vi "ConfigFlattenProgramToXML.vi"(8 "error in (no error)":errorcluster, 11 "ProgramArray":string[][](array[string])) -> (0 "error out":errorcluster, 3 "ProgramXML":string)   [LabVIEW 2018, in "Config.lvlib"]
uses:
  Config.lvlib
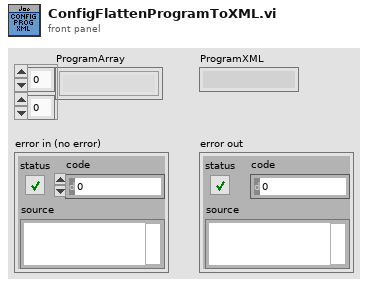
[diagram p1: front panel]
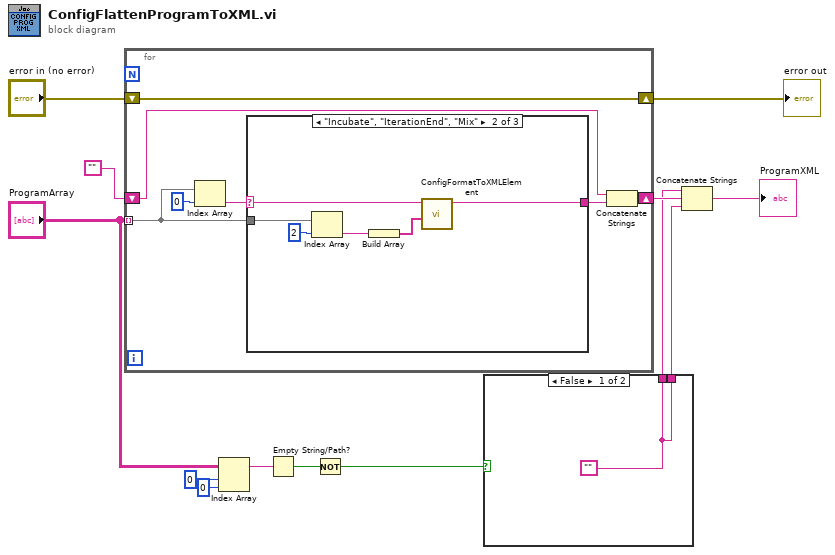
[diagram p0: block diagram]
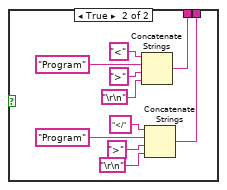
[diagram p2: hidden frame]
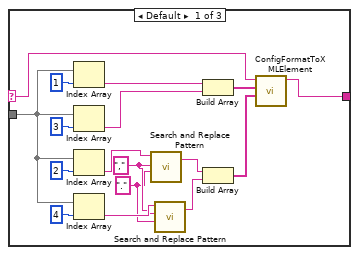
[diagram p3: hidden frame]
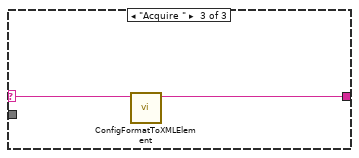
[diagram p4: hidden frame]
diagram:
  n1 = for {
    tunnel: "ProgramArray" -> [w18] mode=indexing
    shift-right: [w16] -> w10
    shift-left: "" -> [w15]
    shift-right: [w14] -> w12
    shift-left: "error in (no error)" -> [w14]
    n2 = Index Array(array=w18, index=0) -> (element=w20:string)
    n3 = case shown="\"Incubate\", \"IterationEnd\", \"Mix\"" w20 {
      selector: w20 -> [w30 w38 w44]
      tunnel: w18 -> [w28 w39 _]
      tunnel: [w27 w40 w45] -> w17
      frame Default {
        w22 = "." ("replace string (\"\")")
        w23 = "," ("regular expression (\"\")")
        n4 = Index Array(array=w28, index=1) -> (element=w34:string)
        n5 = Index Array(array=w28, index=3) -> (element=w33:string)
        n6 = Index Array(array=w28, index=2) -> (element=w26:string)
        n7 = Index Array(array=w28, index=4) -> (element=w24:string)
        n8 = call <vilib>:"Search and Replace Pattern.vi"("string"=w26, "regular expression (\"\")"=w23, "replace string (\"\")"=w22) -> ("result string"=w25:string)  [unwired: 2 in, 1 out]
        n9 = call <vilib>:"Search and Replace Pattern.vi"("string"=w24, "regular expression (\"\")"=w23, "replace string (\"\")"=w22) -> ("result string"=w21:string)  [unwired: 2 in, 1 out]
        n10 = Build Array(w34, w33) -> (w29:string[])
        n11 = Build Array(w25, w21) -> (w37:string[])
        n12 = call "ConfigFormatToXMLElement.vi"("Value"=w37, "Inner Tag"=w29, "outer Tag"=w30) -> ("Resulting String"=w27:string)  [unwired: 8 in]
      }
      frame "Incubate", "IterationEnd", "Mix" {
        n13 = Index Array(array=w39, index=2) -> (element=w42:string)
        n14 = Build Array(w42) -> (w41:string[])
        n15 = call "ConfigFormatToXMLElement.vi"("Value"=w41, "outer Tag"=w38) -> ("Resulting String"=w40:string)  [unwired: 9 in]
      }
      frame "Acquire " {
        n16 = call "ConfigFormatToXMLElement.vi"("outer Tag"=w44) -> ("Resulting String"=w45:string)  [unwired: 10 in]
      }
    }
    n17 = Concatenate Strings(w15, w17) -> (w16:string)
  }
  "error out" <- w12
  n18 = Index Array(array="ProgramArray", index (row)=0 ("disabled index (row)"), index (col)=0 ("disabled index (col)")) -> (element=w4:string)
  n19 = Empty String/Path?(string/path=w4) -> (empty?=w5:bool)
  n20 = Not(x=w5) -> (.not. x?=w1:bool)
  n21 = case shown="False" w1 {
    tunnel: [w46 w55] -> w9
    tunnel: [w46 w54] -> w8
    frame False {
      w46 = ""
    }
    frame True {
      n22 = Concatenate Strings("<" ("string"), "Program" ("string"), ">" ("string"), "\r\n") -> (w54:string)
      n23 = Concatenate Strings("</" ("string"), "Program" ("string"), ">" ("string"), "\r\n") -> (w55:string)
    }
  }
  n24 = Concatenate Strings(w8, w10, w9) -> (→"ProgramXML":string)
